vi "S11 to Z.vi"(8 "Error In":errorcluster, 9 "S11":cdb[](array[numeric]), 10 "Ref. Z [Ohm]":cdb=50.0+0.0i) -> (0 "Error Out":errorcluster, 1 "Z [Ohm]":cdb[](array[numeric]))   [LabVIEW 2016]
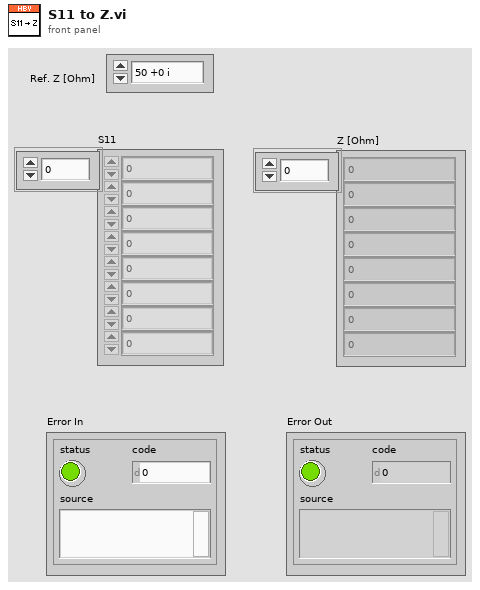
[diagram p1: front panel]
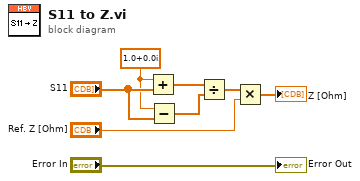
[diagram p0: block diagram]
diagram:
  w3 = cdb 1.0+0.0i
  n1 = Add(x=w3, y="S11") -> (x+y=w7:cdb[])
  n2 = Subtract(x=w3, y="S11") -> (x-y=w4:cdb[])
  n3 = Divide(x=w7, y=w4) -> (x/y=w5:cdb[])
  n4 = Multiply(x=w5, y="Ref. Z [Ohm]") -> (x*y=→"Z [Ohm]":cdb[])
  "Error Out" <- "Error In"
